vi "Percent To Degrees.vi"(1 "Percent":dbl) -> (0 "Degrees":dbl)   [LabVIEW 2016, in "CML UI.lvlib" / "Circular Cue Helper.lvlib"]
uses:
  Circular Cue Helper.lvlib
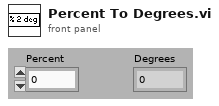
[diagram p1: front panel]
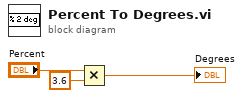
[diagram p0: block diagram]
diagram:
  n1 = Multiply(x="Percent", y=3.6) -> (x*y=→"Degrees":dbl)
